vi "Set Request.vi"(7 "Complete Call (T)":bool=TRUE, 8 "error in (no error)":errorcluster, 10 "package_templatemessage":T1, 11 "gRPCid":T2) -> (0 "error out":errorcluster)   [LabVIEW 2019, in "Generated_server.lvlib"]
uses:
  Generated_server.lvlib
  <vilib>/gRPC/LabVIEW gRPC Library/Shared/grpcId.ctl
  Request.ctl
  Request_request_oneof/Request_request_oneof.lvclass
  Request_Flat.ctl
  Request_request_oneof/Request_request_oneof.lvclass/Request_request_oneof.ctl
  dcc74a39-081a-4bdd-860b-8ed792803c96.vi
  Request_request_oneof/GetActiveFieldIndex.vi
  Request_request_oneof/Getmessage.vi
  Request_request_oneof/Getrequest_id.vi
  <vilib>/gRPC/LabVIEW gRPC Library/Shared/TranslateGrpcError.vi
  <vilib>/gRPC/LabVIEW gRPC Library/Server API/Server/Get Server DLL Path.vi
  <vilib>/Utility/error.llb/Error Cluster From Error Code.vi
  <vilib>/Utility/error.llb/Simple Error Handler.vi
  <vilib>/gRPC/LabVIEW gRPC Library/grpc-lvsupport-release.lvlib
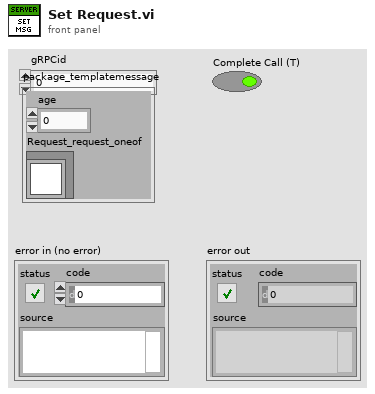
[diagram p1: front panel]
types:
  T1 = typedef "Generated_server.lvlib/Request.ctl" = cluster{"age":i32, "Request_request_oneof":refnum<class "Request_request_oneof.lvclass">}
  T2 = typedef "grpc-lvsupport-release.lvlib/grpcId.ctl" = u64
  T3 = typedef "Generated_server.lvlib/Request_Flat.ctl" = cluster{"age":i32, "Request_request_oneof_selected_index":i32, "message":string, "request_id":i32}
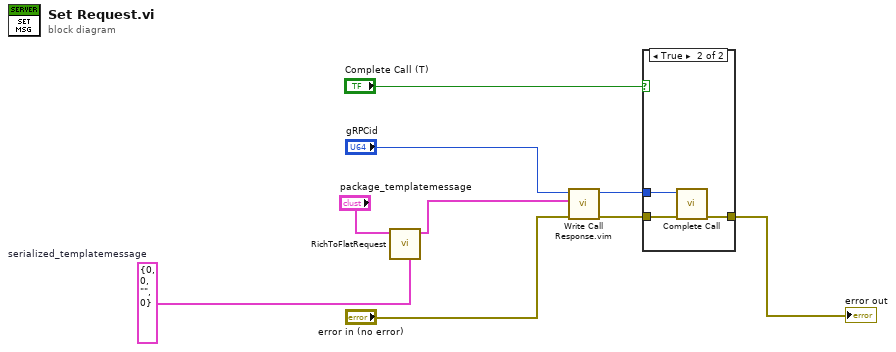
[diagram p0: block diagram]
diagram:
  w2 = T3 {"age"=0, "Request_request_oneof_selected_index"=0, "message"="", "request_id"=0}  # serialized_templatemessage
  n1 = call "RichToFlatRequest.vi"("OutputClusterType"=w2, "InputCluster"="package_templatemessage") -> ("OutputCluster"=w1:T3)  [unwired: 9 in]
  n2 = call "Write Call Response.vim"("error in"="error in (no error)", "Response Data"=w1, "gRPCid in"="gRPCid") -> ("error out"=w6:errorcluster, "gRPCid out"=w7:T2)  [unwired: 7 in]
  n3 = case shown="True" "Complete Call (T)" {
    tunnel: [w10 w13] -> w9
    tunnel: w7 -> [_ w12]
    tunnel: w6 -> [w10 w11]
    frame False {
    }
    frame True {
      n4 = call <vilib>:"Complete Call.vi"("gRPCid"=w12, "error in"=w11) -> ("error out"=w13:errorcluster)  [unwired: 8 in]
    }
  }
  "error out" <- w9
